vi "Update Device list.vi"(8 "MB status":T2 {"MB update(s)" format="%.2g"; "ProCoDA Request"."PC update (s)" format="%.2f"; "ProCoDA Request"."# registers" min=1}, 9 "MB status in":T2[](array[typedef]) {"MB update(s)" format="%.2g"; "ProCoDA Request"."PC update (s)" format="%.2f"; "ProCoDA Request"."# registers" min=1}, 10 "MB ID-Address":T1, 11 "Devices in":T1[](array[typedef])) -> (0 "index":i32, 1 "MB status out":T2[](array[typedef]) {"MB update(s)" format="%.2g"; "ProCoDA Request"."PC update (s)" format="%.2f"; "ProCoDA Request"."# registers" min=1}, 2 "output value":dbl, 3 "Devices out":T1[](array[typedef]))   [LabVIEW 2019]
uses:
  MB status.ctl
  ProCoDA MB Request.ctl
  Read Write.ctl
  MB ID-Address.ctl
panel:
  in  "min update before delete":dbl=10.0
  out "min value":dbl
  out "max value":dbl
  # "s"
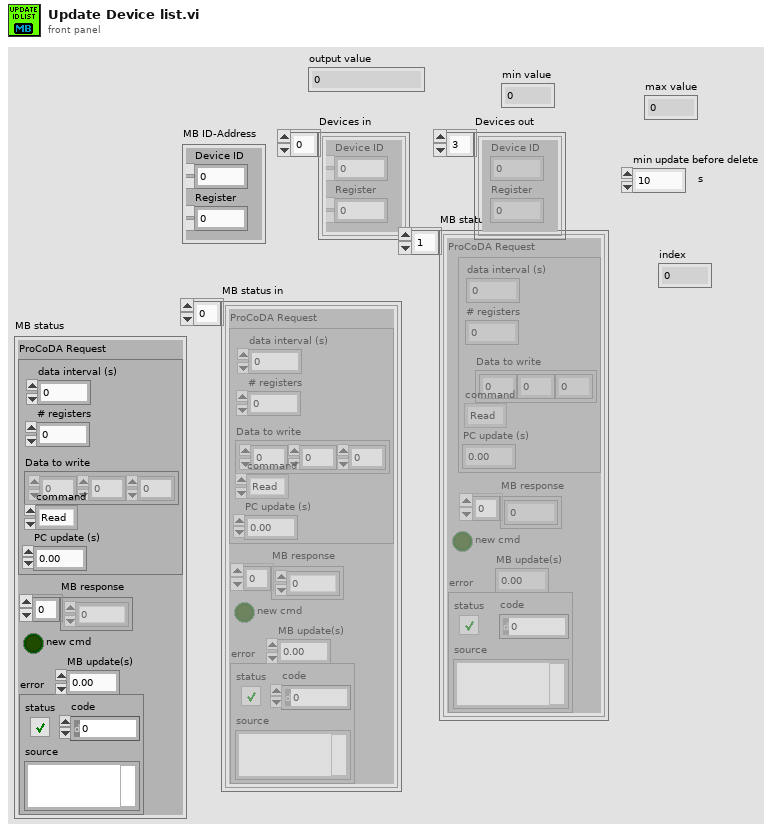
[diagram p1: front panel]
types:
  T1 = typedef "MB ID-Address.ctl" = cluster{"Device ID":u8, "Register":u16}
  T2 = typedef "MB status.ctl" = cluster{"ProCoDA Request":T3, "MB response":dbl[], "new cmd":bool, "error":errorcluster, "MB update(s)":dbl}
  T3 = typedef "ProCoDA MB Request.ctl" = cluster{"# registers":u8, "Data to write":u16[], "data interval (s)":dbl, "command":T4, "PC update (s)":dbl}
  T4 = typedef "Read Write.ctl" = enum16{"Read", "Write"}
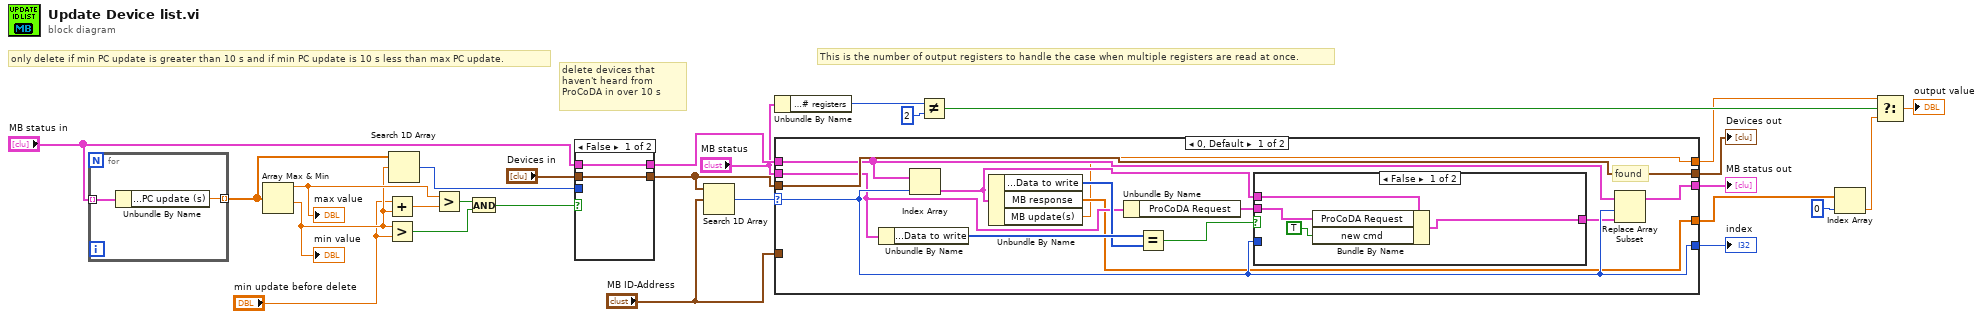
[diagram p0: block diagram]
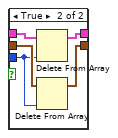
[diagram p2: hidden frame]
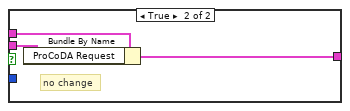
[diagram p3: hidden frame]
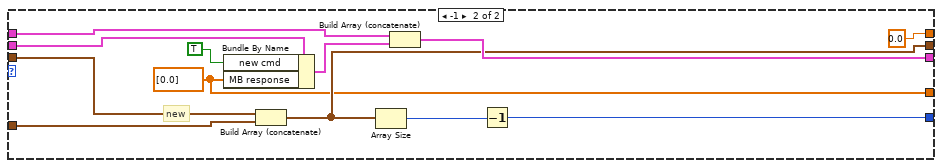
[diagram p4: hidden frame]
diagram:
  # "This is the number of output registers to handle the case when multiple registers are read at once."
  # "only delete if min PC update is greater than 10 s and if min PC update is 10 s less than max PC update."
  # "delete devices that haven't heard from ProCoDA in over 10 s"
  n1 = for {
    tunnel: "MB status in" -> [w29] mode=indexing
    tunnel: [w28] -> w24 mode=indexing
    n2 = Unbundle By Name(w29) -> ("ProCoDA Request.PC update (s)"=w28:dbl)
  }
  n3 = Array Max & Min(array=w24) -> (max value=w25:dbl, min value=w3:dbl)  [unwired: 2 out]
  "max value" <- w25
  "min value" <- w3
  n4 = Add(x="min update before delete", y=w3) -> (x+y=w26:dbl)
  n5 = Greater?(x=w3, y="min update before delete") -> (0:w4:bool)
  n6 = Search 1D Array(1D array=w24, element=w3) -> (index of element=w22:i32)  [unwired: 1 in]
  n7 = Greater?(x=w25, y=w26) -> (0:w6:bool)
  n8 = And(x=w6, y=w4) -> (x .and. y?=w5:bool)
  n9 = case shown="False" w5 {
    tunnel: w22 -> [_ w32]
    tunnel: "Devices in" -> [w31 w36]
    tunnel: [w31 w35] -> w20
    tunnel: "MB status in" -> [w30 w34]
    tunnel: [w30 w33] -> w19
    frame False {
    }
    frame True {
      n10 = Delete From Array(array=w34, index=w32) -> (array with subset deleted=w33:T2[])  [unwired: 1 in, 1 out]
      n11 = Delete From Array(array=w36, index=w32) -> (array with subset deleted=w35:T1[])  [unwired: 1 in, 1 out]
    }
  }
  n12 = Search 1D Array(1D array=w20, element="MB ID-Address") -> (index of element=w27:i32)  [unwired: 1 in]
  n13 = Unbundle By Name("MB status") -> ("ProCoDA Request.# registers"=w8:u8)
  n14 = case shown="0, Default" w27 {
    selector: w27 -> [w47 _]
    tunnel: "MB status" -> [w43 w61]
    tunnel: w19 -> [w41 w66]
    tunnel: [w44 w65] -> w17
    tunnel: [w49 w64] -> w23
    tunnel: w20 -> [w49 w68]
    tunnel: "MB ID-Address" -> [_ w67]
    tunnel: [w47 w62] -> w11
    tunnel: [w39 w58] -> w13
    tunnel: [w37 0.0 ("MB update(s)")] -> w1
    frame 0, Default {
      # "found"
      n15 = Unbundle By Name(w43) -> ("ProCoDA Request.Data to write"=w46:u16[])
      n16 = Index Array(array=w41, index=w47) -> (element=w40:T2)
      n17 = Unbundle By Name(w40) -> ("ProCoDA Request.Data to write"=w45:u16[], "MB response"=w39:dbl[], "MB update(s)"=w37:dbl)
      n18 = Unbundle By Name(w43) -> ("ProCoDA Request"=w38:T3)
      n19 = Equal?(x=w46, y=w45) -> (x = y?=w48:bool)
      n20 = case shown="False" w48 {
        tunnel: w47 -> [_ _]
        tunnel: [w53 w55] -> w42
        tunnel: w40 -> [w51 w56]
        tunnel: w38 -> [w50 w54]
        frame False {
          n21 = Bundle By Name(cluster=w51, "ProCoDA Request"=w50, "new cmd"=TRUE ("new element/subarray")) -> (w53:T2)
        }
        frame True {
          # "no change"
          n22 = Bundle By Name(cluster=w56, "ProCoDA Request"=w54) -> (w55:T2)
        }
      }
      n23 = Replace Array Subset(array=w41, new element=w42, index=w47) -> (w44:T2[])
    }
    frame -1 {
      w58 = dbl[] [0.0]
      # "new"
      n24 = Bundle By Name(cluster=w61, "new cmd"=TRUE ("new element/subarray"), "MB response"=w58) -> (w60:T2)
      n25 = Build Array (concatenate)(w68, w67) -> (w64:T1[])
      n26 = Array Size(array=w64) -> (size(s)=w63:i32)
      n27 = Build Array (concatenate)(w66, w60) -> (w65:T2[])
      n28 = Decrement(x=w63) -> (x-1=w62:i32)
    }
  }
  "MB status out" <- w17
  "Devices out" <- w23
  "index" <- w11
  n29 = Not Equal?(x=w8, y=2) -> (x != y?=w15:bool)
  n30 = Index Array(array=w13, index=0) -> (element=w14:dbl)
  n31 = Select(t=w1, s=w15, f=w14) -> (s? t:f=→"output value":dbl)
